vi "Get Icon Index Over.vi"(7 "UI Mouse Up":bool, 8 "error in (no error)":errorcluster, 10 "Mouse Coordinates":T2, 11 "Toolbar Control in":refnum<class "Toolbar Control.lvclass">) -> (0 "error out":errorcluster, 1 "Button Name":string, 2 "Icon Index Over":i32, 3 "Toolbar Control out":refnum<class "Toolbar Control.lvclass">, 5 "Button State":T1)   [LabVIEW 2011, in "Toolbar Control.lvclass"]
doc: "This Vi will return the information about the icon that the mouse is over. Based on <B>Mouse Coordinates</B>. This may generate a user event stating that a button was clicked if <B>UI Mouse Up</B> is <B>TRUE</B>.\n\n-------------\nDeveloped by Brian Hoover (hooovahh)"
uses:
  Toolbar Control.lvclass
  <vilib>/Utility/miscctls.llb/LVPoint32TypeDef.ctl
  Controls/Button State.ctl
  Toolbar Control.lvclass/Toolbar Control.ctl
  Controls/Button Pressed User Event Data.ctl
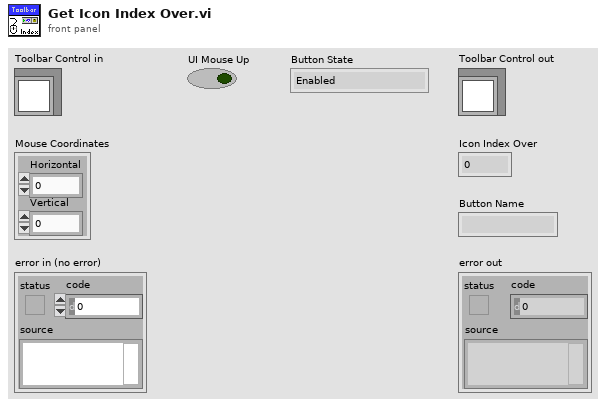
[diagram p1: front panel]
types:
  T1 = typedef "Toolbar Control.lvclass/Button State.ctl" = enum8{"Enabled", "Disabled", "Disabled and Grayed Out"}
  T2 = typedef "LVPoint32TypeDef.ctl" = cluster{"Horizontal":i32, "Vertical":i32}
  T3 = typedef "Button Pressed User Event Data.ctl" = cluster{"Button Pressed":string, "Button State":T1, "Icon Index Over":i32}
  T4 = typedef "Toolbar Control.lvclass/Icon Data.ctl" = cluster{"Original Image Path":path, "Original Image Data":T5, "Scaled Icon":picture, "Button Name":string, "Button State":T1, "Icon Type":T6}
  T5 = typedef "imagedata.ctl" = cluster{"image type":i32, "image depth":i32, "image":u8[], "mask":u8[], "colors":u32[], "Rectangle":cluster{"left":i16, "top":i16, "right":i16, "bottom":i16}}
  T6 = typedef "Icon Type.ctl" = enum16{"Normal Icon", "Separator Icon", "More Options"}
  T7 = typedef "LVRectTypeDef.ctl" = cluster{"Left":i16, "Top":i16, "Right":i16, "Bottom":i16}
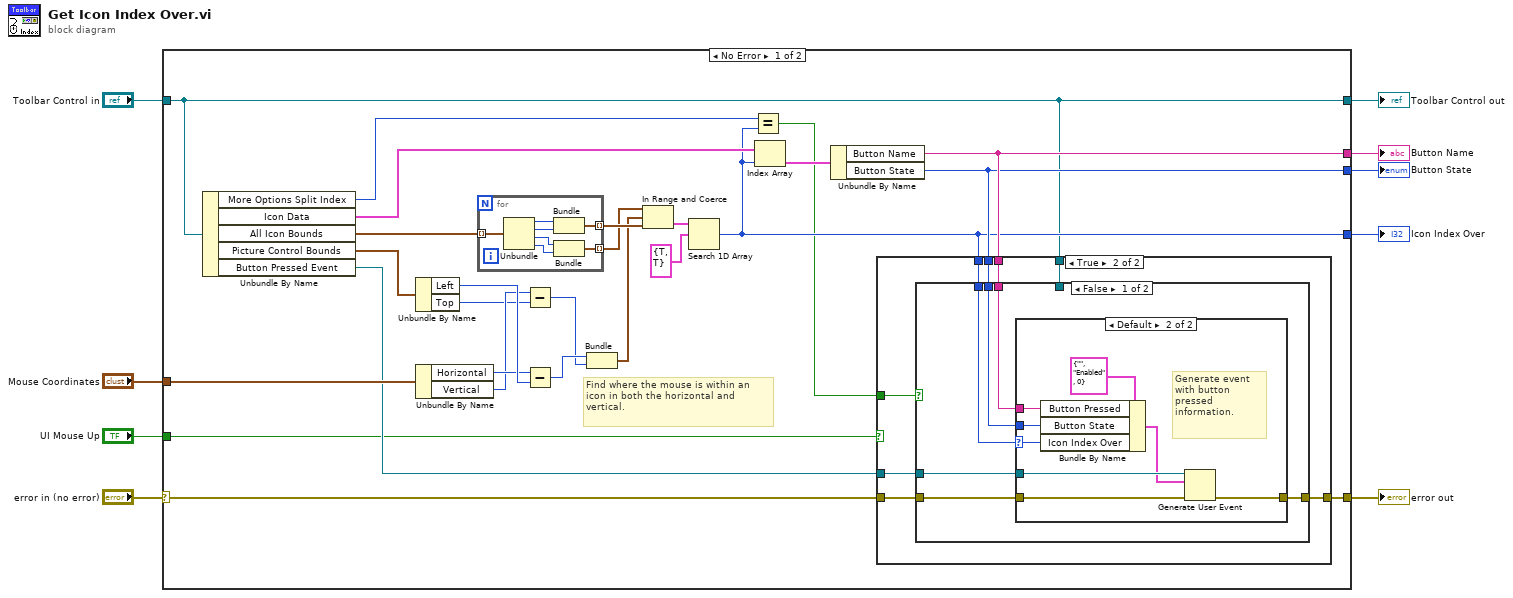
[diagram p0: block diagram]
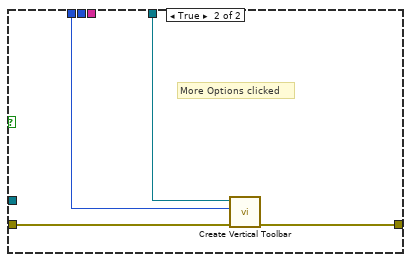
[diagram p4: hidden frame]
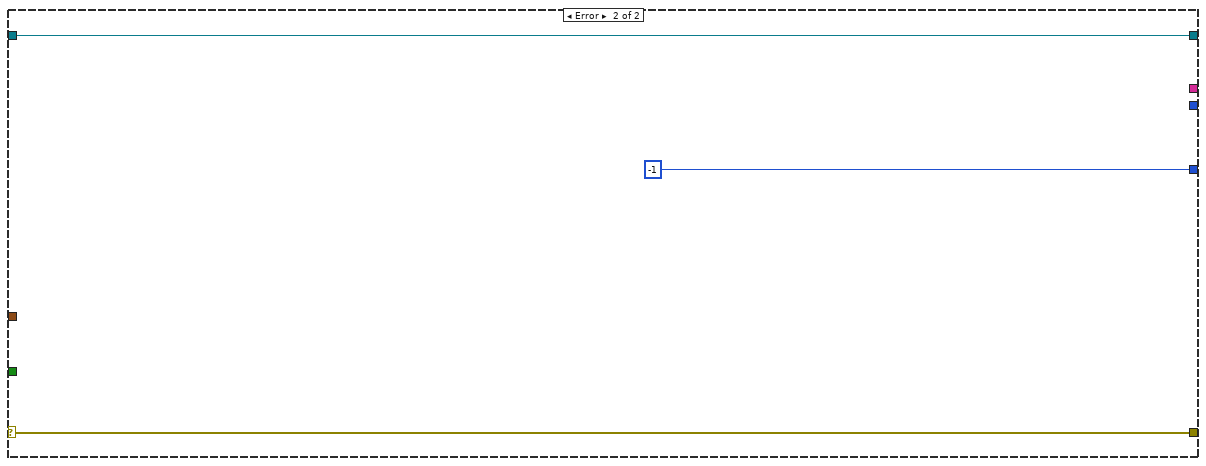
[diagram p5: hidden frame]
diagram:
  n1 = case shown="No Error" "error in (no error)" {
    selector: "error in (no error)" -> [w35 w73]
    tunnel: [w18 w73] -> w8
    tunnel: [w10 w72] -> w6
    tunnel: "Toolbar Control in" -> [w10 w72]
    tunnel: "Mouse Coordinates" -> [w32 _]
    tunnel: [w14 -1 ("index of element")] -> w4
    tunnel: [w16 _] -> w3
    tunnel: [w15 _] -> w2
    tunnel: "UI Mouse Up" -> [w12 _]
    frame No Error {
      # "Find where the mouse is within an icon in both the horizontal and vertical."
      n2 = Unbundle By Name(w10) -> ("More Options Split Index"=w13:i32, "Icon Data"=w20:T4[], "All Icon Bounds"=w29:T7[], "Picture Control Bounds"=w21:T7, "Button Pressed Event"=w17:refnum<user-event>)
      n3 = Unbundle By Name(w21) -> ("Left"=w34:i16, "Top"=w30:i16)
      n4 = Unbundle By Name(w32) -> ("Horizontal"=w33:i32, "Vertical"=w31:i32)
      n5 = for {
        tunnel: w29 -> [w70] mode=indexing
        tunnel: [w65] -> w26 mode=indexing
        tunnel: [w64] -> w25 mode=indexing
        n6 = Unbundle(w70) -> ("Left"=w69:i16, "Top"=w68:i16, "Right"=w67:i16, "Bottom"=w66:i16)
        n7 = Bundle("Left"=w69, "Top"=w68) -> (w65:cluster{"Left":i16, "Top":i16})  [unwired: 1 in]
        n8 = Bundle("Right"=w67, "Bottom"=w66) -> (w64:cluster{"Right":i16, "Bottom":i16})  [unwired: 1 in]
      }
      n9 = Subtract(x=w31, y=w30) -> (x-y=w23:i32)
      n10 = Subtract(x=w33, y=w34) -> (x-y=w24:i32)
      n11 = Bundle(w24, w23) -> (w22:cluster{i32, i32})  [unwired: 1 in]
      n12 = In Range and Coerce(upper limit=w25, x=w22, lower limit=w26) -> (In Range?=w28:cluster{"Left":bool, "Top":bool}[])  [unwired: 1 out]
      n13 = Search 1D Array(1D array=w28, element=cluster{"Right":bool, "Bottom":bool} {"Right"=TRUE, "Bottom"=TRUE}) -> (index of element=w14:i32)  [unwired: 1 in]
      n14 = Equal?(x=w13, y=w14) -> (x = y?=w11:bool)
      n15 = Index Array(array=w20, index=w14) -> (element=w19:T4)
      n16 = Unbundle By Name(w19) -> ("Button Name"=w16:string, "Button State"=w15:T1)
      n17 = case shown="True" w12 {
        tunnel: w35 -> [w36 w44]
        tunnel: [w36 w43] -> w18
        tunnel: w17 -> [_ w42]
        tunnel: w16 -> [_ w41]
        tunnel: w15 -> [_ w40]
        tunnel: w14 -> [_ w39]
        tunnel: w11 -> [_ w38]
        tunnel: w10 -> [_ w37]
        frame False {
        }
        frame True {
          n18 = case shown="False" w38 {
            tunnel: w44 -> [w50 w62]
            tunnel: [w49 w61] -> w43
            tunnel: w42 -> [w48 _]
            tunnel: w41 -> [w47 _]
            tunnel: w40 -> [w46 _]
            tunnel: w39 -> [w45 w60]
            tunnel: w37 -> [_ w63]
            frame False {
              n19 = case shown="Default" w45 {
                selector: w45 -> [_ w52]
                tunnel: w50 -> [w51 w59]
                tunnel: [w51 w58] -> w49
                tunnel: w48 -> [_ w57]
                tunnel: w47 -> [_ w54]
                tunnel: w46 -> [_ w53]
                frame -1 {
                }
                frame Default {
                  # "Generate event with button pressed information."
                  n20 = Bundle By Name(cluster=T3 {"Button Pressed"="", "Button State"=enum."Enabled", "Icon Index Over"=0} ("Button Pressed"), "Button Pressed"=w54, "Button State"=w53, "Icon Index Over"=w52) -> (w55:T3)
                  n21 = Generate User Event(user event=w57, event data cluster=w55, error in=w59) -> (error out=w58:errorcluster)  [unwired: 1 out]
                }
              }
            }
            frame True {
              # "More Options clicked"
              n22 = call "Create Vertical Toolbar.vi"("error in (no error)"=w62, "Button Over Index"=w60, "Toolbar Control in"=w63) -> ("error out"=w61:errorcluster)  [unwired: 8 in]
            }
          }
        }
      }
    }
    frame Error {
    }
  }
  "error out" <- w8
  "Toolbar Control out" <- w6
  "Icon Index Over" <- w4
  "Button Name" <- w3
  "Button State" <- w2
